vi "PPLVI.vi"(11 "Numeric":dbl) -> (3 "Numeric 2":dbl)   [LabVIEW 2017, in "PPL.lvlib"]
uses:
  PPL.lvlib
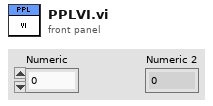
[diagram p1: front panel]
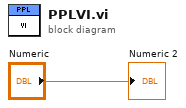
[diagram p0: block diagram]
diagram:
  "Numeric 2" <- "Numeric"
